vi "LDA_analogue_start_time_sync_PN.vi"(4 "Correlation peak fit method":enum32{"Max", "Quadratic", "Gaussian"}(ring)=enum."Quadratic", 5 "Pulse high threshold (Volts)":dbl=2.5, 6 "Analogue dt (s)":dbl, 7 "Analogue LDA burst pulse array":dbl[](array[numeric]), 8 "LDA arrival Times":dbl[](array[numeric])) -> (1 "valid bursts checksum status":bool=TRUE, 2 "Absolute LDA times (s)":dbl[](array[numeric]), 3 "LDA start time rel. to Analogue (s)":dbl)   [LabVIEW 2013]
uses:
  <vilib>/Analysis/1siggen.llb/Ramp Pattern by Samples.vi
  <vilib>/Analysis/2dsp.llb/1D Cross Correlation (DBL).vi
  <vilib>/Analysis/polynomials.llb/Polynomial Roots (DBL).vi
  <vilib>/Analysis/polynomials.llb/nth Derivative of Polynomial (DBL).vi
  <vilib>/Analysis/NI_AALPro.lvlib
  <vilib>/Analysis/NI_AALBase.lvlib
panel:
  out "Xcorr LDA timings":cluster{"Ramp Pattern":dbl[], dbl[]}[](graph)
  in  "Pts. either side of peak to use in fit":i32=3
  out "Analogue LDA burst pulse array":cluster{"index (row)":dbl, dbl, "Vout":dbl[]}(graph)
  out "Thresholded LDA burst times (valid only)":cluster{"index (row)":dbl, dbl, "Vout":dbl[]}(graph)
  out "Thresholded LDA arr time checksum":i32
  out "Thresholded LDA burst times (valid + invalid)":cluster{"index (row)":dbl, dbl, "Vout":dbl[]}(graph)
  out "LDA counted pulses (valid + invalid)":i32
  out "LDA arr_t length":i32
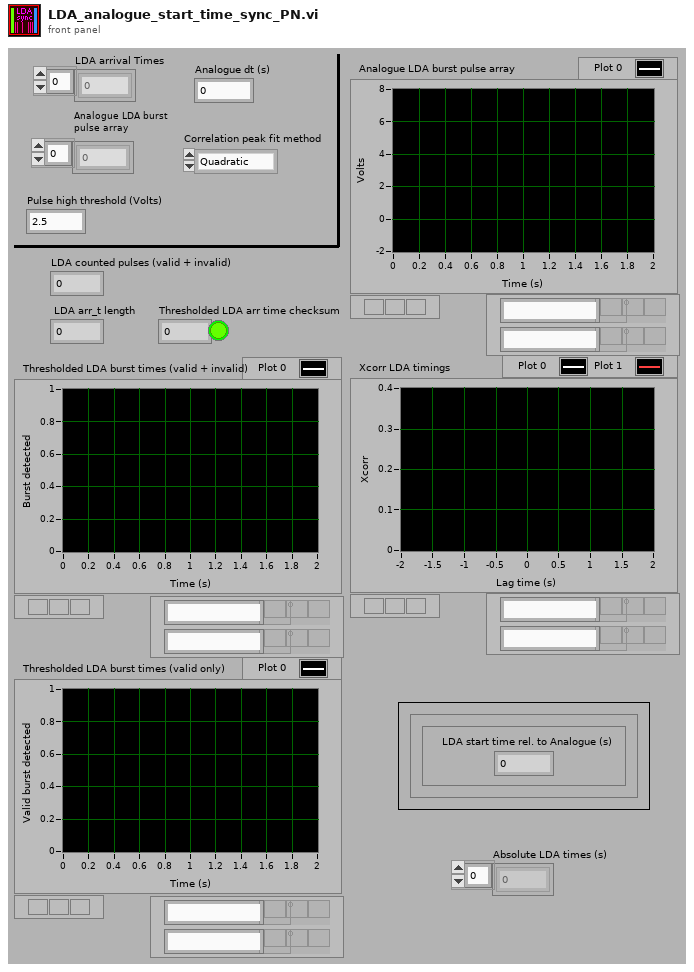
[diagram p1: front panel]
types:
  T1 = cluster{"index (row)":dbl, "Analogue dt (s)":dbl, "Vout":dbl[]}
  T2 = cluster{"index (row)":dbl, "Analogue dt (s)":dbl, "Analogue LDA burst pulse array":dbl[]}
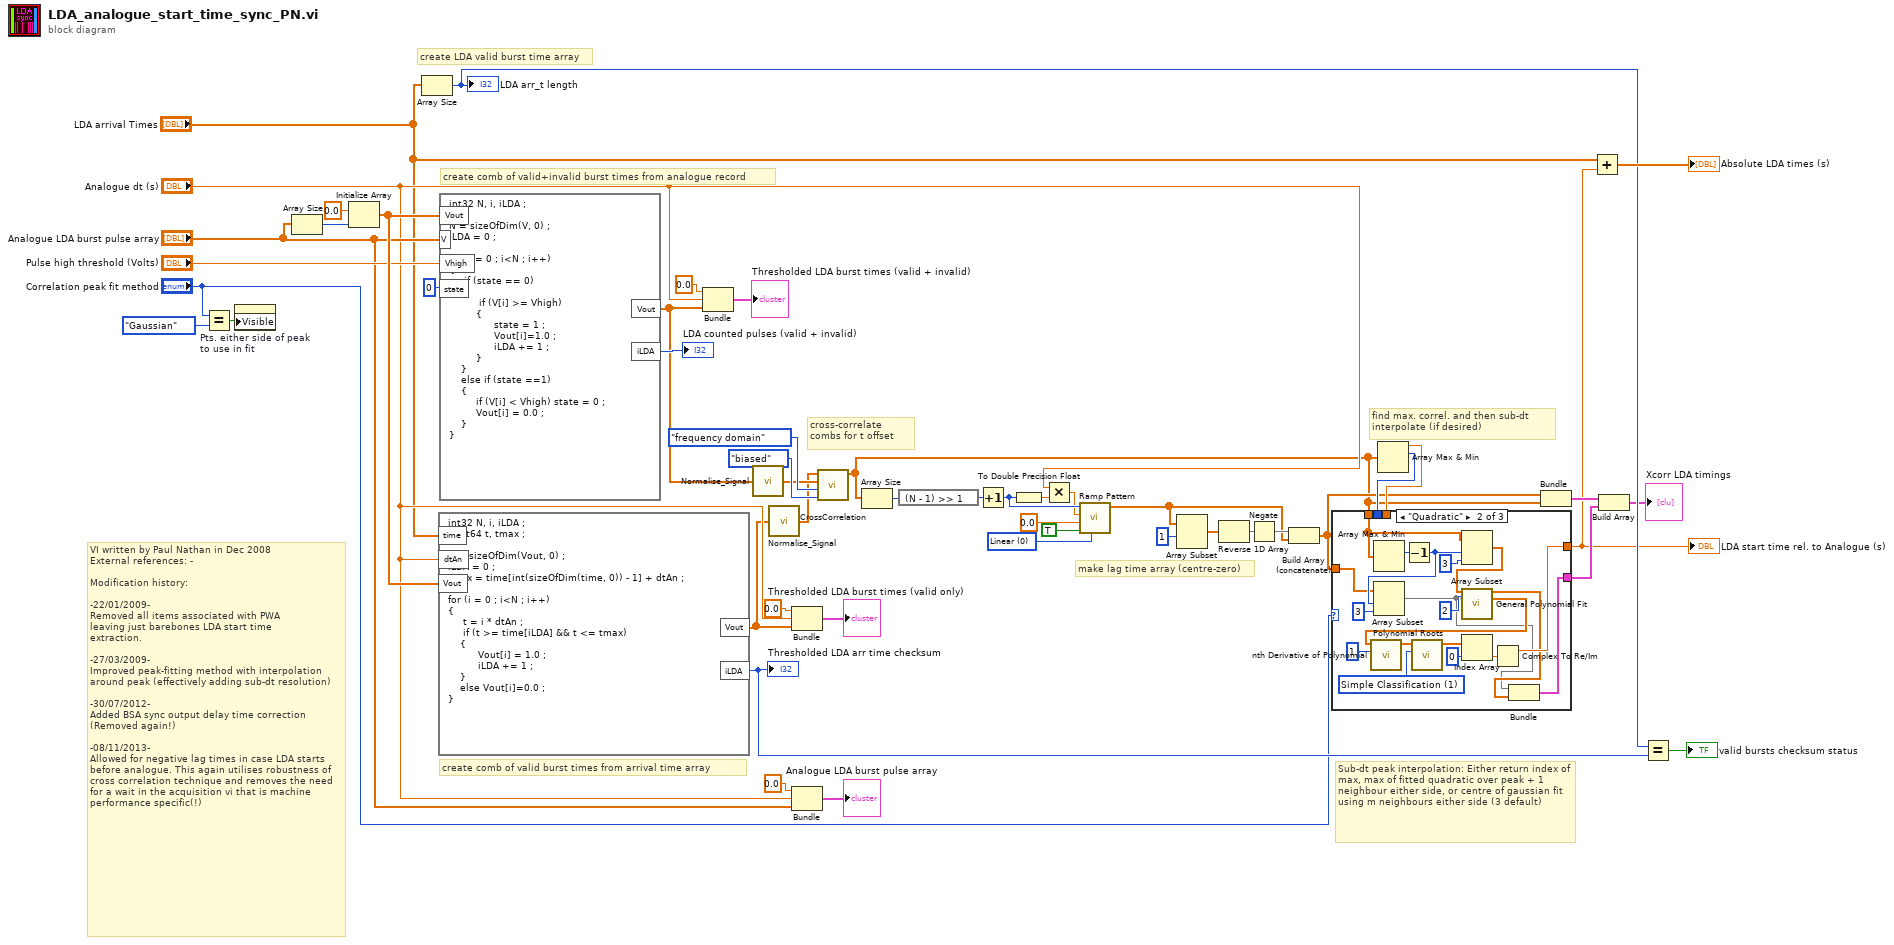
[diagram p0: block diagram]
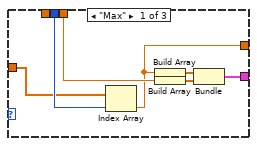
[diagram p2: hidden frame]
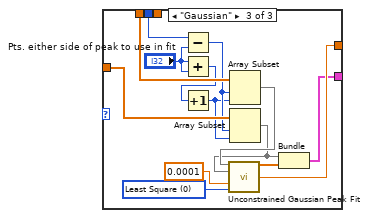
[diagram p3: hidden frame]
diagram:
  w20 = u16 0 items=["Linear", "Logarithmic"] ("type")
  # "make lag time array (centre-zero)"
  # "find max. correl. and then sub-dt interpolate (if desired)"
  # "Sub-dt peak interpolation: Either return index of max, max of fitted quadratic over peak + 1 neighbour either side, or centre of gaussian fit using m neighbours either side (3 default)"
  # "create LDA valid burst time array"
  # "cross-correlate combs for t offset"
  # "VI written by Paul Nathan in Dec 2008\nExternal references: -\n\nModification history:\n\n-22/01/2009-\nRemoved all items associated with PWA\nleaving just barebones LDA start time\nextraction.\n\n-27/03/2009-\nImproved peak-fitting method with interpolation around peak (effectively adding sub-dt resolution)\n\n-30/07/2012-\nAdded BSA sync output delay time correction\n(Removed again!)\n\n-08/11/2013-\nAllowed for negative lag times in case LDA starts before analogue. This again utilises robustness of cross correlation technique and removes the need for a wait in the acquisition vi that is machine performance specific(!)"
  # "create comb of valid+invalid burst times from analogue record"
  # "create comb of valid burst times from arrival time array"
  n1 = Equal?(x="Correlation peak fit method", y=enum32{"Max", "Quadratic", "Gaussian"}."Gaussian") -> (x = y?=w15:bool)
  n2 = property on="Pts. either side of peak to use in fit" class="DigNum (strict)"("Visible"=w15) -> ()  [unwired: 2 in, 2 out]
  n3 = Array Size(array="Analogue LDA burst pulse array") -> (size(s)=w40:i32)
  n4 = Initialize Array(0.0 ("element"), w40) -> (w39:dbl[])
  n5 = Array Size(array="LDA arrival Times") -> (size(s)=w35:i32)
  "LDA arr_t length" <- w35
  n6 = formula code="int32 N, i, iLDA ;\nfloat64 t, tmax ;\n\nN = sizeOfDim(Vout, 0) ;\niLDA = 0 ;\ntmax = time[int(sizeOfDim(time, 0)) - 1] + dtAn ;\n\nfor (i = 0 ; i<N ; i++)\n{\n     t = i * dtAn ;\n     if (t >= time[iLDA] && t <= tmax) \n    {\n          Vout[i] = 1.0 ;\n          iLDA += 1 ;\n    }\n    else Vout[i]=0.0 ;\n}"("dtAn"="Analogue dt (s)", "time"="LDA arrival Times", "Vout"=w39) -> ("Vout"=w10:dbl[], "iLDA"=w38:i32)
  "Thresholded LDA arr time checksum" <- w38
  n7 = formula code="int32 N, i, iLDA ;\n\nN = sizeOfDim(V, 0) ;\niLDA = 0 ;\n\nfor (i = 0 ; i<N ; i++)\n{\n     if (state == 0) \n    {\n          if (V[i] >= Vhigh)\n         {\n               state = 1 ;\n               Vout[i]=1.0 ;\n               iLDA += 1 ;\n         }\n    }\n    else if (state ==1)\n    {\n         if (V[i] < Vhigh) state = 0 ;\n         Vout[i] = 0.0 ;\n    }\n}"("V"="Analogue LDA burst pulse array", "Vhigh"="Pulse high threshold (Volts)", "state"=u8 0 ("input variable"), "Vout"=w39) -> ("Vout"=w12:dbl[], "iLDA"=→"LDA counted pulses (valid + invalid)":i32)
  n8 = Bundle("index (row)"=0.0, "Analogue dt (s)"="Analogue dt (s)", "Vout"=w12) -> (→"Thresholded LDA burst times (valid + invalid)":T1)  [unwired: 1 out]
  n9 = call "Normalise_Signal.vi"("x"=w12) -> ("(x-X)/sigma"=w11:dbl[])  [unwired: 4 in]
  n10 = call "Normalise_Signal.vi"("x"=w10) -> ("(x-X)/sigma"=w9:dbl[])  [unwired: 4 in]
  n11 = Bundle("index (row)"=0.0, "Analogue dt (s)"="Analogue dt (s)", "Vout"=w10) -> (→"Thresholded LDA burst times (valid only)":T1)  [unwired: 1 out]
  n12 = Bundle("index (row)"=0.0, "Analogue dt (s)"="Analogue dt (s)", "Analogue LDA burst pulse array"="Analogue LDA burst pulse array") -> (→"Analogue LDA burst pulse array":T2)  [unwired: 1 out]
  n13 = call-poly <vilib>:"CrossCorrelation.vi"("normalization"=enum32{"none", "unbiased", "biased"}."biased", "algorithm"=enum32{"direct", "frequency domain"}."frequency domain", "Y"=w11, "X"=w9) -> ("Rxy"=w4:dbl[])  [unwired: 7 out]
  n14 = Array Size(array=w4) -> (size(s)=w41:i32)
  n15 = expression code="(N - 1) >> 1"(w41) -> (w22:i32)
  n16 = Increment(x=w22) -> (x+1=w29:i32)
  n17 = To Double Precision Float(number=w29) -> (double precision float=w27:dbl)
  n18 = Multiply(x="Analogue dt (s)", y=w27) -> (x*y=w28:dbl)
  n19 = call-poly <vilib>:"Ramp Pattern.vi"("type"=w20, "exclude end?"=TRUE, "start"=0.0, "end"=w28, "samples"=w29) -> ("Ramp Pattern"=w3:dbl[])  [unwired: 5 in, 1 out]
  n20 = Array Subset(array=w3, index=1) -> (w2:dbl[])  [unwired: 1 in]
  n21 = Reverse 1D Array(array=w2) -> (reversed array=w7:dbl[])
  n22 = Negate(x=w7) -> (-x=w6:dbl[])
  n23 = Build Array (concatenate)(w6, w3) -> (w5:dbl[])
  n24 = Array Max & Min(array=w4) -> (max value=w18:dbl, max index (indices)=w19:i32)  [unwired: 2 out]
  n25 = case shown="\"Quadratic\"" "Correlation peak fit method" {
    tunnel: w4 -> [_ w64 w86]
    tunnel: [w50 w65 w88] -> w13
    tunnel: [w56 w62 w78] -> w17
    tunnel: w5 -> [w51 w58 w83]
    tunnel: w19 -> [w52 _ w85]
    tunnel: w18 -> [w53 _ _]
    frame "Max" {
      n26 = Index Array(array=w51, index=w52) -> (element=w50:dbl)
      n27 = Build Array(w50) -> (w54:dbl[])
      n28 = Build Array(w53) -> (w55:dbl[])
      n29 = Bundle(w54, w55) -> (w56:cluster{dbl[], dbl[]})  [unwired: 1 out]
    }
    frame "Quadratic" {
      w69 = u16 1 items=["General", "Simple Classification", "Refinement", "Advanced Refinement"] ("option")
      n30 = Array Max & Min(array=w64) -> (max index (indices)=w74:i32)  [unwired: 3 out]
      n31 = Decrement(x=w74) -> (x-1=w59:i32)
      n32 = Array Subset(array=w58, index=w59, length=3) -> (w57:dbl[])
      n33 = Array Subset(array=w64, index=w59, length=3) -> (w73:dbl[])
      n34 = call <vilib>:"General Polynomial Fit.vi"("Y"=w73, "polynomial order"=2, "X"=w57) -> ("Best Polynomial Fit"=w61:dbl[], "Polynomial Coefficients"=w63:dbl[])  [unwired: 9 in, 2 out]
      n35 = call-poly <vilib>:"nth Derivative of Polynomial.vi"("order"=1, "P(x)"=w63) -> ("Nth Derivative of P(x)"=w70:dbl[])  [unwired: 9 out]
      n36 = call-poly <vilib>:"Polynomial Roots.vi"("option"=w69, "P(x)"=w70) -> ("Roots"=w68:cdb[])  [unwired: 9 out]
      n37 = Index Array(array=w68, index=0) -> (element=w66:cdb)
      n38 = Complex To Re/Im(x + iy=w66) -> (x=w65:dbl)  [unwired: 1 out]
      n39 = Bundle(w57, "Best Polynomial Fit"=w61) -> (w62:cluster{dbl[], "Best Polynomial Fit":dbl[]})  [unwired: 1 out]
    }
    frame "Gaussian" {
      w87 = u16 0 items=["Least Square", "Least Absolute Residual", "Bisquare"] ("method")
      n40 = Subtract(x=w85, y="Pts. either side of peak to use in fit") -> (x-y=w82:i32)
      n41 = Add(x="Pts. either side of peak to use in fit", y="Pts. either side of peak to use in fit") -> (x+y=w76:i32)
      n42 = Increment(x=w76) -> (x+1=w77:i32)
      n43 = Array Subset(array=w86, index=w82, length=w77) -> (w81:dbl[])
      n44 = Array Subset(array=w83, index=w82, length=w77) -> (w79:dbl[])
      n45 = call <vilib>:"Unconstrained Gaussian Peak Fit.vi"("Y"=w81, "X"=w79, "tolerance"=0.0001, "method"=w87) -> ("Best Gaussian Fit"=w80:dbl[], "center"=w88:dbl)  [unwired: 6 in, 4 out]
      n46 = Bundle(w79, "Best Gaussian Fit"=w80) -> (w78:cluster{dbl[], "Best Gaussian Fit":dbl[]})  [unwired: 1 out]
    }
  }
  "LDA start time rel. to Analogue (s)" <- w13
  n47 = Bundle(w5, "Rxy"=w4) -> (w23:cluster{dbl[], "Rxy":dbl[]})  [unwired: 1 out]
  n48 = Add(x="LDA arrival Times", y=w13) -> (x+y=→"Absolute LDA times (s)":dbl[])
  n49 = Build Array(w23, w17) -> (→"Xcorr LDA timings":cluster{dbl[], "Best Gaussian Fit":dbl[]}[])
  n50 = Equal?(x=w35, y=w38) -> (x = y?=→"valid bursts checksum status":bool)
